vi "UDP Named Service - Client.vi"() -> ()   [LabVIEW 2025]
doc: "This VI implements a client for the UDP Named Service - Server.vi. It connects to a service by specifying the server address and the name of the service. The client receives the string sent by the server, displays the string and closes the connection.\nAuthor: Scott Hannahs <sth@magnet.fsu.edu>\n\nThis software is licensed for use under the “MIT License\"\nCopyright (c) 2025 Scott Hannahs, sth@sth@magnet.sthnet.net\n\nPermission is hereby granted, free of charge, to any person obtaining a copy of this software and associated documentation files (the \"Software\"), to deal in the Software without restriction, including without limitation the rights to use, copy, modify, merge, publish, distribute, sublicense, and/or sell copies of the Software, and to permit persons to whom the Software is furnished to do so, subject to the following conditions: The above copyright notice and this permission notice shall be included in all copies or substantial portions of the Software.\n\nTHE SOFTWARE IS PROVIDED \"AS IS\", WITHOUT WARRANTY OF ANY KIND, EXPRESS OR IMPLIED, INCLUDING BUT NOT LIMITED TO THE WARRANTIES OF MERCHANTABILITY, FITNESS FOR A PARTICULAR PURPOSE AND NONINFRINGEMENT. IN NO EVENT SHALL THE AUTHORS OR COPYRIGHT HOLDERS BE LIABLE FOR ANY CLAIM, DAMAGES OR OTHER LIABILITY, WHETHER IN AN ACTION OF CONTRACT, TORT OR OTHERWISE, ARISING FROM, OUT OF OR IN CONNECTION WITH THE SOFTWARE OR THE USE OR OTHER DEALINGS IN THE SOFTWARE."
panel:
  out "name":string
  out "Remote port":u16
  out "Local port":u16
  in  "Command":string="status"
  out "Message from Server":string
  # "Overview: Demonstrates the use of the UDP functions to connect to a UDP server VI via named service and receive data.\nInstructions:\n1. Ensure UDP Named Service - Server.vi is already running.\n2. Run the VI."
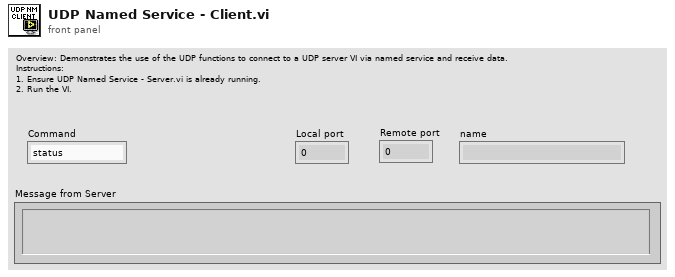
[diagram p1: front panel]
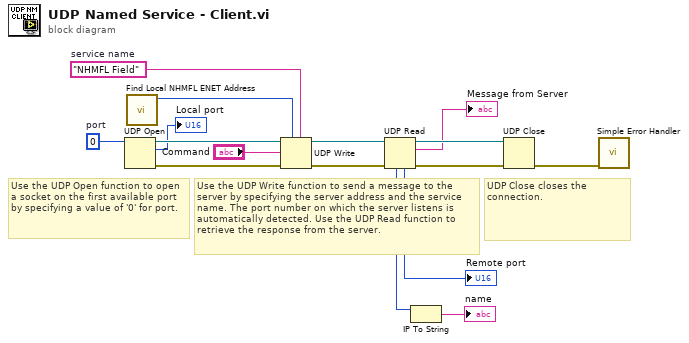
[diagram p0: block diagram]
diagram:
  w2 = "NHMFL Field"  # service name
  w13 = u16 0  # port
  # "UDP Close closes the connection."
  # "Use the UDP Open function to open a socket on the first available port by specifying a value of '0' for port."
  # "Use the UDP Write function to send a message to the server by specifying the server address and the service name. The port number on which the server listens is automatically detected. Use the UDP Read function to retrieve the response from the server."
  n1 = UDP Open(11:w13) -> (port=w15:refnum<k16>, 0:w16:errorcluster, 2:→"Local port":u16)  [unwired: 4 in]
  n2 = call "Find Local NHMFL ENET Address.vi"() -> ("Ethernet Address"=w1:u32)  [unwired: 9 in, 2 out]
  n3 = UDP Write(address=w1, port or service name=w2, connection ID=w15, data in="Command", 8:w16) -> (error out=w12:errorcluster, 3:w11:refnum<k16>)  [unwired: 1 in]
  n4 = UDP Read(connection ID=w11, 8:w12) -> (data out=→"Message from Server":string, error out=w9:errorcluster, 3:w10:refnum<k16>, 4:→"Remote port":u16, 6:w5:u32)  [unwired: 2 in]
  n5 = IP To String(2:w5) -> (0:→"name":string)  [unwired: 1 in]
  n6 = UDP Close(connection ID=w10, 8:w9) -> (error out=w14:errorcluster)  [unwired: 1 out]
  n7 = call <vilib>:"Simple Error Handler.vi"("error in (no error)"=w14) -> ()  [unwired: 4 in, 5 out]
